vi "lib Match Files in Folder.vi"(8 "error in (no error)":errorcluster, 10 "Reg Ex":string[](array[string]), 11 "Folder":path) -> (0 "error out":errorcluster, 3 "Matching Files":string[](array[string]))   [LabVIEW 2011]
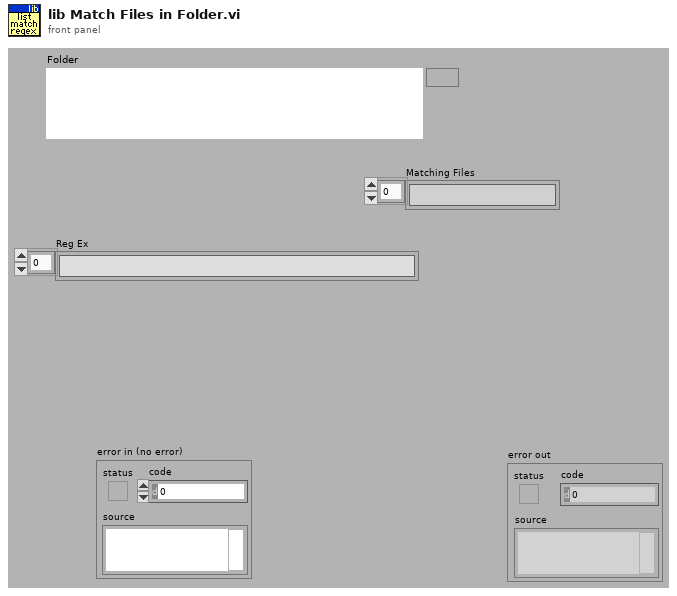
[diagram p1: front panel]
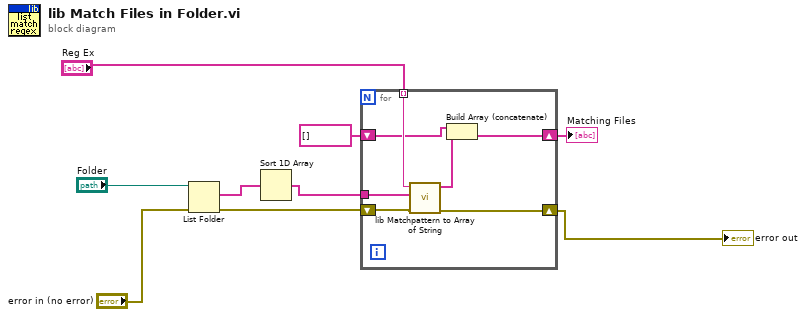
[diagram p0: block diagram]
diagram:
  n1 = List Folder(path="Folder", error in="error in (no error)") -> (filenames=w8:string[], error out=w9:errorcluster)  [unwired: 2 in, 2 out]
  n2 = Sort 1D Array(array=w8) -> (sorted array=w7:string[])
  n3 = for {
    tunnel: "Reg Ex" -> [w15] mode=indexing
    tunnel: w7 -> [w14]
    shift-right: [w11] -> w1
    shift-left: string[] [] -> [w10]
    shift-right: [w13] -> w2
    shift-left: w9 -> [w16]
    n4 = call "lib Matchpattern to Array of String.vi"("error in (no error)"=w16, "filenames"=w14, "Pattern"=w15) -> ("error out"=w13:errorcluster, "Matches"=w12:string[])  [unwired: 7 in]
    n5 = Build Array (concatenate)(w10, w12) -> (w11:string[])
  }
  "error out" <- w2
  "Matching Files" <- w1
